vi "TestExec.Config, Get Facility Name and Location.vi"(8 "error in (no error)":errorcluster, 11 "Config File":path) -> (0 "error out":errorcluster, 2 "Location":string, 3 "Name":string)   [LabVIEW 2018]
uses:
  <vilib>/Utility/config.llb/Read Key (String).vi
  <vilib>/Utility/config.llb/NI_LVConfig.lvlib
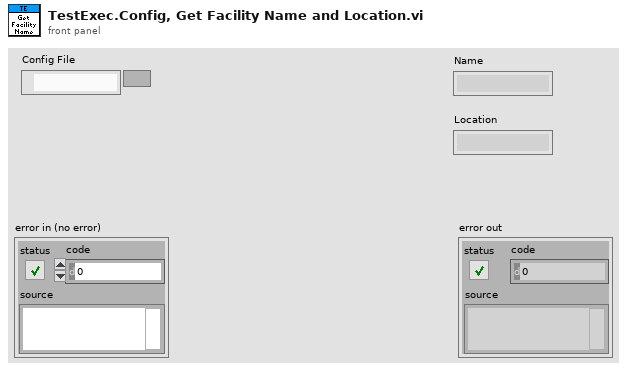
[diagram p1: front panel]
types:
  T1 = typedef "NI_LVConfig.lvlib/Config Data RefNum.ctl" = refnum<k1>
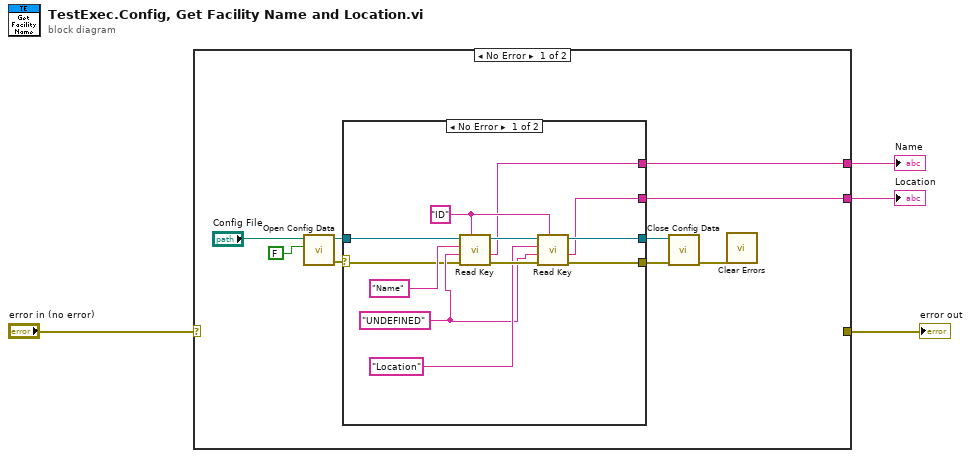
[diagram p0: block diagram]
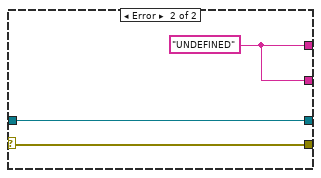
[diagram p2: hidden frame]
diagram:
  n1 = case shown="No Error" "error in (no error)" {
    selector: "error in (no error)" -> [_ w29]
    tunnel: [_ w29] -> w3
    tunnel: [w8 _] -> w2
    tunnel: [w7 _] -> w1
    frame No Error {
      n2 = call <vilib>:"Open Config Data.vi"("create file if necessary (T)"=FALSE, "configuration file path"="Config File") -> ("error out"=w5:errorcluster, "refnum"=w12:T1)  [unwired: 7 in, 1 out]
      n3 = case shown="No Error" w5 {
        selector: w5 -> [w14 w26]
        tunnel: w12 -> [w23 w27]
        tunnel: [w19 w27] -> w10
        tunnel: [w18 w26] -> w9
        tunnel: [w17 w28] -> w8
        tunnel: [w16 w28] -> w7
        frame No Error {
          w15 = "UNDEFINED"
          w21 = "ID"
          n4 = call-poly <vilib>:"Read Key.vi"("section"=w21, "error in (no error)"=w14, "default value"=w15, "key"="Name", "refnum"=w23) -> ("error out"=w22:errorcluster, "value"=w16:string, "refnum out"=w24:T1)  [unwired: 3 in, 1 out]
          n5 = call-poly <vilib>:"Read Key.vi"("section"=w21, "error in (no error)"=w22, "default value"=w15, "key"="Location", "refnum"=w24) -> ("error out"=w18:errorcluster, "value"=w17:string, "refnum out"=w19:T1)  [unwired: 3 in, 1 out]
        }
        frame Error {
          w28 = "UNDEFINED"
        }
      }
      n6 = call <vilib>:"Close Config Data.vi"("error in (no error)"=w9, "refnum"=w10) -> ("error out"=w13:errorcluster)  [unwired: 8 in, 1 out]
      n7 = call <vilib>:"Clear Errors.vi"("error in (no error)"=w13) -> ()  [unwired: 5 in, 2 out]
    }
    frame Error {
    }
  }
  "error out" <- w3
  "Name" <- w1
  "Location" <- w2
